vi "server_pos_indicator.vi"(5 "reset":bool, 7 "rough":bool, 8 "error in":errorcluster, 10 "yc":dbl, 11 "xc":dbl) -> (0 "error out":errorcluster)   [LabVIEW 2014]
panel:
  out "rough Array":bool[](array[boolean])
  out "rough":i32
  out "size(s)":i32
  out "output array":T1(array[cluster])
  out "position":picture
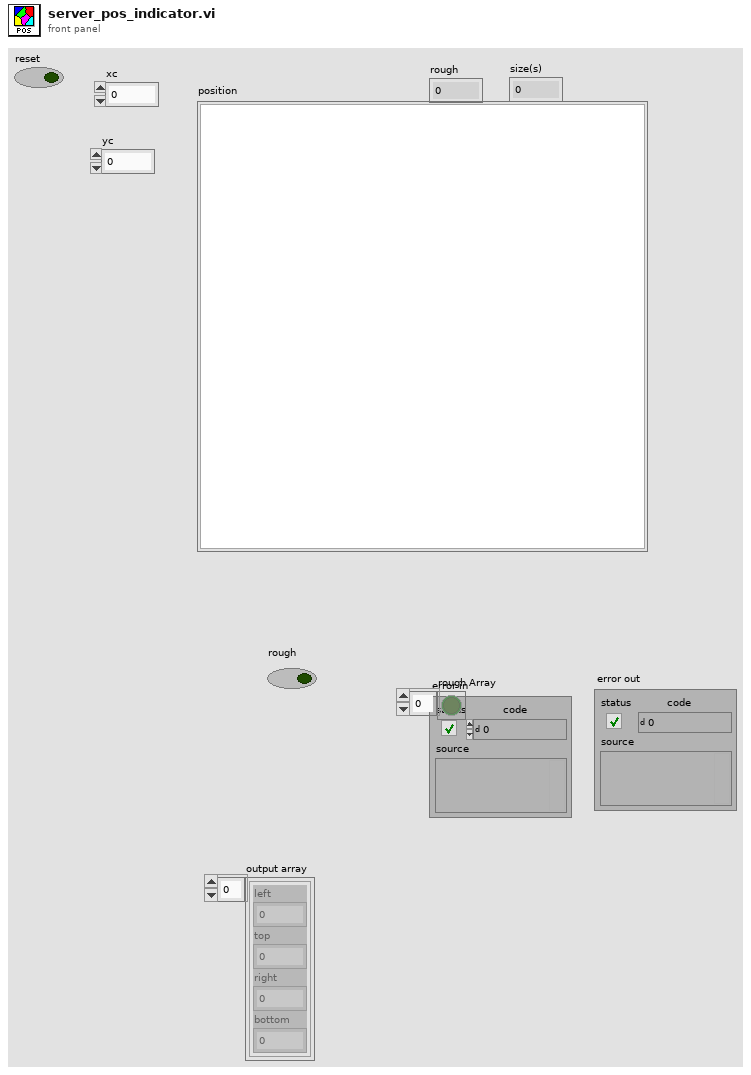
[diagram p1: front panel]
types:
  T1 = cluster{"left":i16, "top":i16, "right":i16, "bottom":i16}[]
  T2 = cluster{"horizontal":enum16{"left", "center", "right"}, "vertical":enum16{"top", "center", "bottom"}}
  T3 = cluster{"left":i16, "top":i16, "right":i16, "bottom":i16}
  T4 = cluster{"Width":u16, "Style":enum32{"Solid", "Dash", "Dot", "DashDot", "DashDotDot"}}
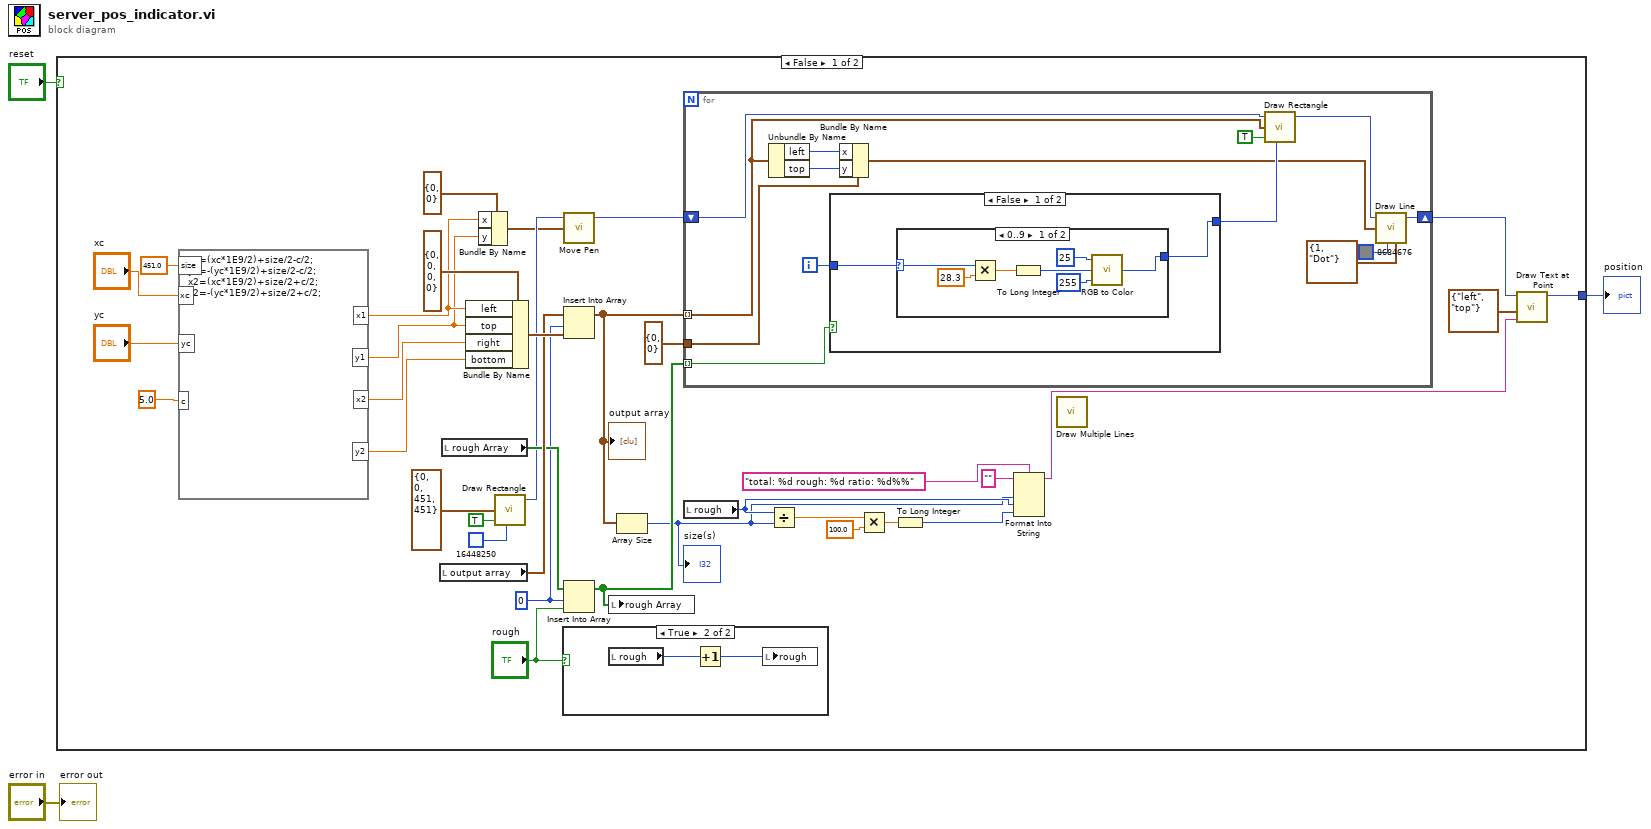
[diagram p0: block diagram]
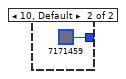
[diagram p3: hidden frame]
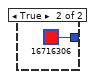
[diagram p4: hidden frame]
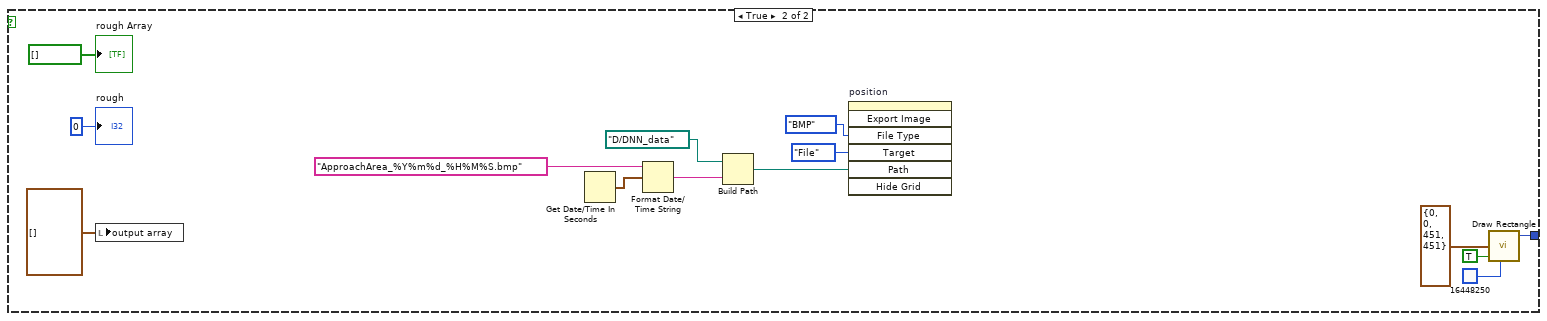
[diagram p5: hidden frame]
diagram:
  n1 = case shown="False" "reset" {
    tunnel: [w13 w76] -> w2
    frame False {
      w23 = 0 ("index")
      n2 = formula code="x1=(xc*1E9/2)+size/2-c/2;\ny1=-(yc*1E9/2)+size/2-c/2;\nx2=(xc*1E9/2)+size/2+c/2;\ny2=-(yc*1E9/2)+size/2+c/2;"("xc"="xc", "yc"="yc", "c"=5.0 ("input variable"), "size"=451.0 ("input variable")) -> ("x1"=w5:dbl, "y1"=w4:dbl, "x2"=w35:dbl, "y2"=w34:dbl)
      n3 = local read "output array"() -> (w27:T1)
      n4 = local read "rough Array"() -> (w26:bool[])
      n5 = Bundle By Name(cluster=T3 {"left"=0, "top"=0, "right"=0, "bottom"=0} ("rect"), "left"=w5, "top"=w4, "right"=w35, "bottom"=w34) -> (w29:T3)
      n6 = Bundle By Name(cluster=cluster{"x":i16, "y":i16} {"x"=0, "y"=0} ("end point"), "x"=w5, "y"=w4) -> (w7:cluster{"x":i16, "y":i16})
      n7 = call <vilib>:"Draw Rectangle.vi"("rect"=T3 {"left"=0, "top"=0, "right"=451, "bottom"=451}, "fill?(F)"=TRUE, "color(black)"=u32 16448250) -> ("new picture"=w9:picture)  [unwired: 6 in]
      n8 = case shown="True" "rough" {
        frame False {
        }
        frame True {
          n9 = local read "rough"() -> (w41:i32)
          n10 = Increment(x=w41) -> (x+1=w40:i32)
          n11 = local write "rough"(w40) -> ()
        }
      }
      n12 = call <vilib>:"Move Pen.vi"("new position"=w7, "picture"=w9) -> ("new picture"=w8:picture)  [unwired: 3 in]
      n13 = Insert Into Array(array=w27, index=w23, new element=w29) -> (w28:T1)
      "output array" <- w28
      n14 = Insert Into Array(array=w26, index=w23, new element="rough") -> (w25:bool[])
      n15 = local write "rough Array"(w25) -> ()
      n16 = Array Size(array=w28) -> (size(s)=w12:i32)
      "size(s)" <- w12
      n17 = for {
        shift-right: [w44] -> w14
        shift-left: w8 -> [w55]
        tunnel: w28 -> [w50] mode=indexing
        tunnel: w25 -> [w51] mode=indexing
        tunnel: cluster{"x":i16, "y":i16} {"x"=0, "y"=0} ("end point") -> [w48]
        i -> [w54]
        n18 = Unbundle By Name(w50) -> ("left"=w47:i16, "top"=w46:i16)
        n19 = case shown="False" w51 {
          tunnel: w54 -> [w57 _]
          tunnel: [w56 u32 16716306 ("color(black)")] -> w52
          frame False {
            n20 = case shown="0..9" w57 {
              selector: w57 -> [w61 _]
              tunnel: [w64 u32 7171459 ("color(black)")] -> w56
              frame 0..9 {
                n21 = Multiply(x=w61, y=28.3) -> (x*y=w63:dbl)
                n22 = To Long Integer(number=w63) -> (32bit integer=w62:i32)
                n23 = call <vilib>:"RGB to Color.vi"("B"=u8 255 ("R"), "G"=w62, "R"=u8 25 ("B")) -> ("Color"=w64:u32)
              }
              frame 10, Default {
              }
            }
          }
          frame True {
          }
        }
        n24 = Bundle By Name(cluster=w48, "x"=w47, "y"=w46) -> (w49:cluster{"x":i16, "y":i16})
        n25 = call <vilib>:"Draw Rectangle.vi"("picture"=w55, "rect"=w50, "fill?(F)"=TRUE, "color(black)"=w52) -> ("new picture"=w45:picture)  [unwired: 5 in]
        n26 = call <vilib>:"Draw Line.vi"("picture"=w45, "end point"=w49, "color(black)"=u32 8684676, "pen"=T4 {"Width"=1, "Style"=enum."Dot"}) -> ("new picture"=w44:picture)  [unwired: 5 in]
      }
      n27 = local read "rough"() -> (w15:i32)
      n28 = Divide(x=w15, y=w12) -> (x/y=w20:dbl)
      n29 = Multiply(x=w20, y=100.0) -> (x*y=w18:dbl)
      n30 = To Long Integer(number=w18) -> (32bit integer=w17:i32)
      n31 = Format Into String(format string="total: %d rough: %d ratio: %d%%", initial string="", w12, w15, w17) -> (resulting string=w16:string)  [unwired: 1 in, 1 out]
      n32 = call <vilib>:"Draw Multiple Lines.vi"() -> ()  [unwired: 9 in, 1 out]
      n33 = call <vilib>:"Draw Text at Point.vi"("text"=w16, "alignment(left, top)"=T2 {"horizontal"=enum."left", "vertical"=enum."top"}, "picture"=w14) -> ("new picture"=w13:picture)  [unwired: 7 in, 1 out]
    }
    frame True {
      n34 = local write "output array"(T1 [] ("output array")) -> ()
      n35 = Get Date/Time In Seconds() -> (seconds since 1Jan1904=w74:timestamp)
      n36 = Format Date/Time String(time format string (%c)="ApproachArea_%Y%m%d_%H%M%S.bmp", seconds (now)=w74) -> (date/time string=w73:string)  [unwired: 1 in]
      n37 = Build Path(base path=path "D:/DNN_data" ("Path"), name or relative path=w73) -> (appended path=w69:path)
      n38 = invoke on="position" class="Pict" method="Export Image"("File Type"=enum32{"BMP", "EPS", "EMF", "PICT"}."BMP", "Target"=enum32{"File", "Clipboard"}."File", "Path"=w69) -> ()  [unwired: 4 in, 7 out]
      n39 = call <vilib>:"Draw Rectangle.vi"("rect"=T3 {"left"=0, "top"=0, "right"=451, "bottom"=451}, "fill?(F)"=TRUE, "color(black)"=u32 16448250) -> ("new picture"=w76:picture)  [unwired: 6 in]
      "rough" <- 0 ("rough")
      "rough Array" <- bool[] []
    }
  }
  "position" <- w2
  "error out" <- "error in"
